vi "Get Icon Body Text.vi"(8 "error in (no error)":errorcluster, 11 "VI Path":string) -> (0 "error out":errorcluster, 2 "Body Text":T1 {"Body Text Spec"."Alignment" items=["left", "center", "right"]}, 3 "VI Path (dup)":string)   [LabVIEW 2013]
uses:
  <vilib>/LabVIEW Icon API/lv_icon/Controls/BodyText.ctl
  <vilib>/LabVIEW Icon API/lv_icon/Controls/Font.ctl
  <vilib>/LabVIEW Icon API/lv_icon/Controls/Alignment.ctl
  <vilib>/LabVIEW Icon API/lv_icon/Classes/Icon/Icon.lvclass
  <vilib>/LabVIEW Icon API/lv_icon/Classes/Icon Framework/Icon Framework.lvclass
  <vilib>/LabVIEW Icon API/LabVIEW Icon API.lvlib
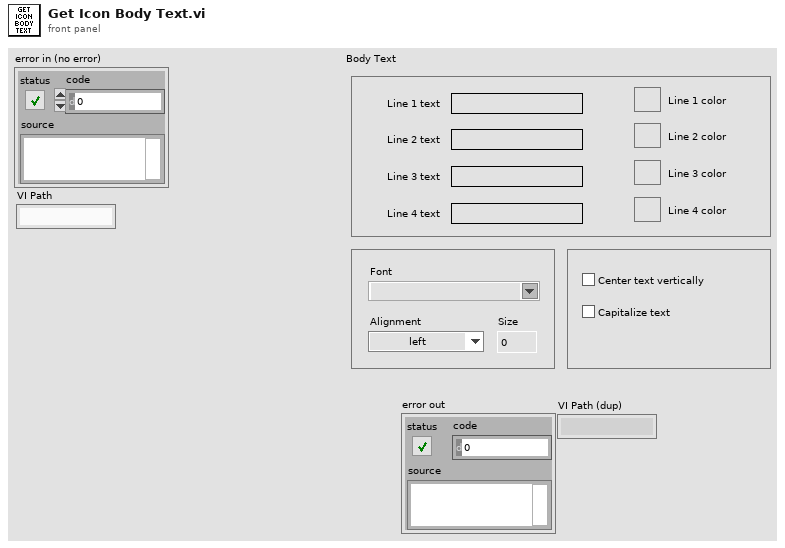
[diagram p1: front panel]
types:
  T1 = typedef "BodyText.ctl" = cluster{"Line 1 text":string, "Line 2 text":string, "Line 3 text":string, "Line 4 text":string, "Line 1 color":u32, "Line 2 color":u32, "Line 3 color":u32, "Line 4 color":u32, "Body Text Spec":cluster{"Font":T2, "Alignment":T3, "Size":u8}, "Center text vertically":bool, "Capitalize Text":bool}
  T2 = typedef "Font.ctl" = string
  T3 = typedef "Alignment.ctl" = u16
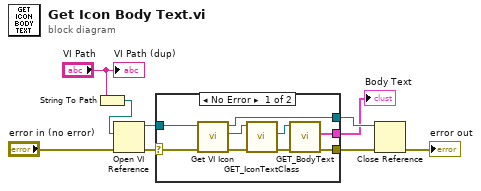
[diagram p0: block diagram]
diagram:
  n1 = String To Path(string="VI Path") -> (path=w1:path)
  n2 = Open VI Reference(vi path=w1, error in (no error)="error in (no error)") -> (vi reference=w8:refnum<vi>, error out=w9:errorcluster)  [unwired: 4 in]
  n3 = case shown="No Error" w9 {
    selector: w9 -> [w17 w19]
    tunnel: w8 -> [w18 w20]
    tunnel: [w14 w19] -> w5
    tunnel: [w13 w20] -> w7
    tunnel: [w10 _] -> w6
    frame No Error {
      n4 = call <vilib>:"Get VI Icon.vi"("error in (no error)"=w17, "VI Refnum in"=w18) -> ("error out"=w16:errorcluster, "Icon"=w12:refnum<class "Icon.lvclass">, "VI Refnum out"=w13:refnum<vi>)  [unwired: 7 in]
      n5 = call-dynamic "GET_IconTextClass.vi"("error in (no error)"=w16, "Icon.lvclass in"=w12) -> ("error out"=w15:errorcluster, "Icon Framework.lvclass"=w11:refnum<class "Icon Framework.lvclass">)  [unwired: 8 out]
      n6 = call-dynamic "GET_BodyText.vi"("error in (no error)"=w15, "Icon Framework.lvclass in"=w11) -> ("error out"=w14:errorcluster, "Body Text"=w10:T1)  [unwired: 6 in, 2 out]
    }
    frame Error {
    }
  }
  "Body Text" <- w6
  n7 = Close Reference(reference=w7, error in (no error)=w5) -> (error out=→"error out":errorcluster)
  "VI Path (dup)" <- "VI Path"
